vi "GetStatus.vi"(8 "error in (no error)":errorcluster) -> (0 "error out":errorcluster)   [LabVIEW 2018, in "LibTiePie.lvlib"]
uses:
  LibTiePie.lvlib
  LabViewHS4/libtiepie.dll
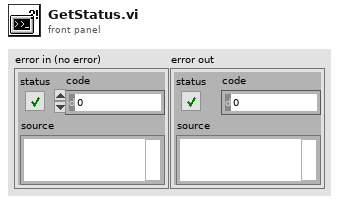
[diagram p1: front panel]
types:
  T1 = cluster{"status":bool, "return type":i32, "return type":string}
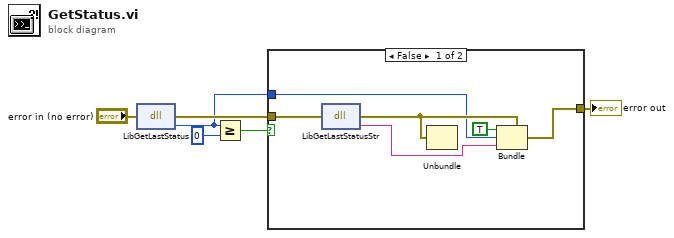
[diagram p0: block diagram]
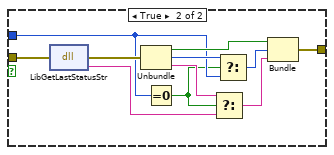
[diagram p2: hidden frame]
diagram:
  n1 = dll-call lib="C:/Users/cwaha/Documents/LabViewHS4/libtiepie.dll" fn="LibGetLastStatus"(error in="error in (no error)") -> (error out=w3:errorcluster, "return type"=w1:i32)  [unwired: 2 in, 1 out]
  n2 = Greater Or Equal?(x=w1, y=0) -> (x >= y?=w4:bool)
  n3 = case shown="False" w4 {
    tunnel: w3 -> [w11 w13]
    tunnel: [w9 w15] -> w2
    tunnel: w1 -> [w7 w17]
    frame False {
      n4 = dll-call lib="C:/Users/cwaha/Documents/LabViewHS4/libtiepie.dll" fn="LibGetLastStatusStr"(error in=w11) -> (error out=w10:errorcluster, "return type"=w8:string)  [unwired: 2 in, 1 out]
      n5 = Unbundle(w10) -> ()  [unwired: 3 out]
      n6 = Bundle(cluster=w10, "status"=TRUE, "code"=w7, "source"=w8) -> (w9:errorcluster)
    }
    frame True {
      n7 = dll-call lib="C:/Users/cwaha/Documents/LabViewHS4/libtiepie.dll" fn="LibGetLastStatusStr"(error in=w13) -> (error out=w23:errorcluster, "return type"=w14:string)  [unwired: 2 in, 1 out]
      n8 = Unbundle(w23) -> ("status"=w22:bool, "code"=w18:i32, "source"=w21:string)
      n9 = Equal To 0?(x=w17) -> (x = 0?=w16:bool)
      n10 = Select(t=w21, s=w16, f=w14) -> (s? t:f=w20:string)
      n11 = Select(t=w18, s=w16, f=w17) -> (s? t:f=w19:i32)
      n12 = Bundle("status"=w22, "return type"=w19, "return type"=w20) -> (w15:T1)  [unwired: 1 in]
    }
  }
  "error out" <- w2
